vi "MultiAxisPositioning.vi"(8 "error in":errorcluster, 10 "Input":T2={"set1"=TRUE, "set2"=TRUE, "set3"=TRUE, "target1"=0, "target2"=0, "target3"=0}, 11 "connection ID":refnum<k5>) -> (0 "error out":errorcluster, 2 "results":T1, 3 "connection ID":refnum<k5>)   [LabVIEW 2016, in "AMC_VIs.lvlib"]
doc: "Simultaneously set 3 axes positions\n and get positions to minimize network latency"
uses:
  AMC_VIs.lvlib
panel:
  out "params_cluster":T2
  in  "Params_cluster":T3
  in  "results_cluster":T4
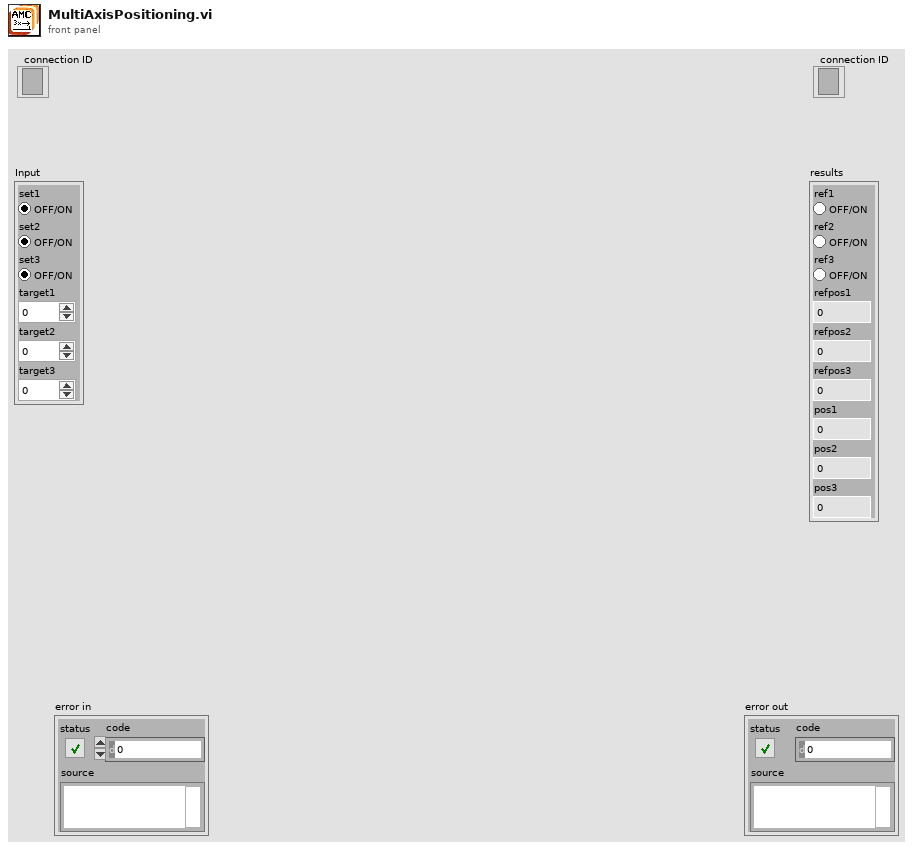
[diagram p1: front panel]
types:
  T1 = cluster{"ref1":bool, "ref2":bool, "ref3":bool, "refpos1":i32, "refpos2":i32, "refpos3":i32, "pos1":i32, "pos2":i32, "pos3":i32}
  T2 = cluster{"set1":bool, "set2":bool, "set3":bool, "target1":i32, "target2":i32, "target3":i32}
  T3 = cluster{"boolean":bool, "boolean":bool, "boolean":bool, "integer":i32, "integer":i32, "integer":i32}
  T4 = cluster{"errNo":i32, "ref1":bool, "ref2":bool, "ref3":bool, "refpos1":i32, "refpos2":i32, "refpos3":i32, "pos1":i32, "pos2":i32, "pos3":i32}
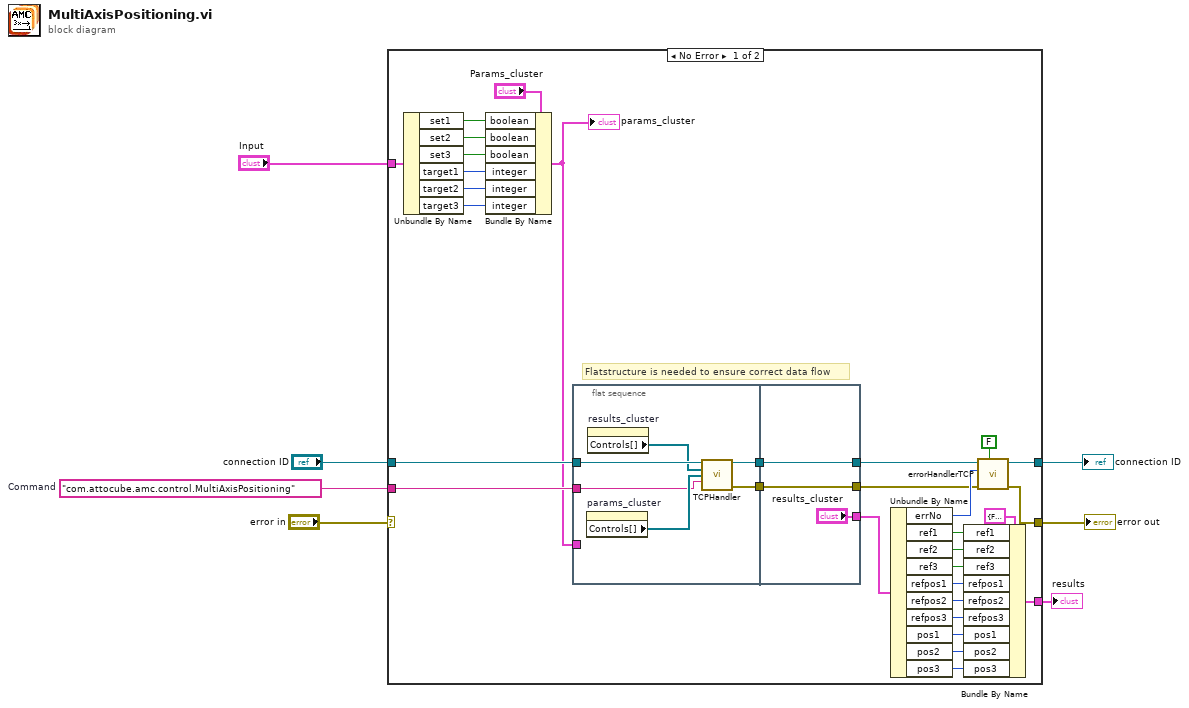
[diagram p0: block diagram]
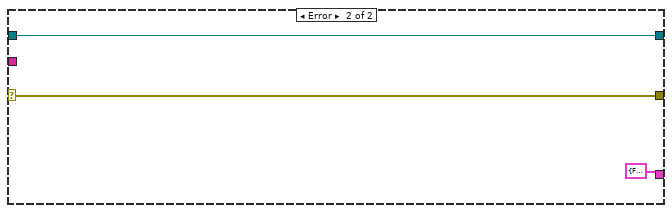
[diagram p2: hidden frame]
diagram:
  w3 = "com.attocube.amc.control.MultiAxisPositioning"  # Command
  n1 = case shown="No Error" "error in" {
    selector: "error in" -> [_ w50]
    tunnel: [w36 w50] -> w7
    tunnel: [w38 w49] -> w6
    tunnel: "connection ID" -> [w35 w49]
    tunnel: w3 -> [w29 _]
    tunnel: "Input" -> [w25 _]
    tunnel: [w8 T1 {"ref1"=FALSE, "ref2"=FALSE, "ref3"=FALSE, "refpos1"=0, "refpos2"=0, "refpos3"=0, "pos1"=0, "pos2"=0, "pos3"=0} ("results_cluster")] -> w1
    frame No Error {
      # "Flatstructure is needed to ensure correct data flow"
      n2 = Unbundle By Name(w25) -> ("set1"=w24:bool, "set2"=w23:bool, "set3"=w22:bool, "target1"=w21:i32, "target2"=w20:i32, "target3"=w19:i32)
      n3 = Bundle By Name(cluster="Params_cluster", "boolean"=w24, "boolean"=w23, "boolean"=w22, "integer"=w21, "integer"=w20, "integer"=w19) -> (w26:T3)
      "params_cluster" <- w26
      n4 = flat-sequence {
        tunnel: [w43] -> w31
        tunnel: w35 -> [w44]
        tunnel: w29 -> [w40]
        tunnel: [w39] -> w27
        tunnel: w26 -> [_]
        tunnel: ["results_cluster"] -> w32
        tunnel: [w47] -> w34
        tunnel: w31 -> [w47]
        tunnel: [w45] -> w28
        tunnel: w27 -> [w45]
        frame #0 {
          n5 = property on="params_cluster" class="Clust (strict)"() -> ("Controls[]"=w41:refnum<vi>[])  [unwired: 2 in, 2 out]
          n6 = property on="results_cluster" class="Clust (strict)"() -> ("Controls[]"=w42:refnum<vi>[])  [unwired: 2 in, 2 out]
          n7 = call "TCPHandler.vi"("connection ID"=w44, "results_cluster"=w42, "params_cluster"=w41, "method"=w40) -> ("connection ID"=w43:refnum<k5>, "error"=w39:errorcluster)  [unwired: 8 in, 2 out]
        }
        frame #1 {
        }
      }
      n8 = Unbundle By Name(w32) -> ("errNo"=w33:i32, "ref1"=w17:bool, "ref2"=w16:bool, "ref3"=w15:bool, "refpos1"=w14:i32, "refpos2"=w13:i32, "refpos3"=w12:i32, "pos1"=w11:i32, "pos2"=w10:i32, "pos3"=w9:i32)
      n9 = Bundle By Name(cluster=T1 {"ref1"=FALSE, "ref2"=FALSE, "ref3"=FALSE, "refpos1"=0, "refpos2"=0, "refpos3"=0, "pos1"=0, "pos2"=0, "pos3"=0} ("results_cluster"), "ref1"=w17, "ref2"=w16, "ref3"=w15, "refpos1"=w14, "refpos2"=w13, "refpos3"=w12, "pos1"=w11, "pos2"=w10, "pos3"=w9) -> (w8:T1)
      n10 = call "errorHandlerTCP.vi"("show popup"=FALSE, "error in"=w28, "error number"=w33, "connection ID"=w34) -> ("error out"=w36:errorcluster, "connection ID"=w38:refnum<k5>)  [unwired: 6 in]
    }
    frame Error {
    }
  }
  "error out" <- w7
  "connection ID" <- w6
  "results" <- w1
